vi "CS++UserContent.vi"   [LabVIEW 2013]
doc: "Place actor and class constants that should be included included in an application on the blockdiagramm."
panel:
  # "Place actor and class constants on the blockdiagramm."
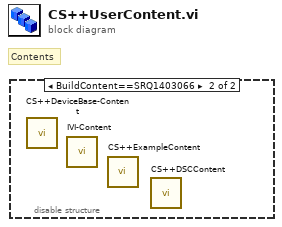
[diagram p0: block diagram]
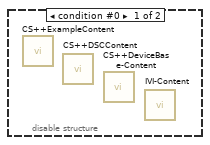
[diagram p2: hidden frame]
diagram:
  # "Contents"
  n1 = disable-structure shown="BuildContent==SRQ1403066" {
    frame condition #0 {
      n2 = call "CS++ExampleContent.vi"() -> ()  [unwired: 12 in]
      n3 = call "CS++DSCContent.vi"() -> ()  [unwired: 12 in]
      n4 = call "CS++DeviceBase-Content.vi"() -> ()  [unwired: 12 in]
      n5 = call "IVI-Content.vi"() -> ()  [unwired: 12 in]
    }
    frame condition #1 (active) {
      n6 = call "CS++DeviceBase-Content.vi"() -> ()  [unwired: 12 in]
      n7 = call "IVI-Content.vi"() -> ()  [unwired: 12 in]
      n8 = call "CS++ExampleContent.vi"() -> ()  [unwired: 12 in]
      n9 = call "CS++DSCContent.vi"() -> ()  [unwired: 12 in]
    }
  }
